vi "ep_Config Info to Task.vi"(6 "trigger timestamp":timestamp, 7 "record info":T1={"station name"="", "recording device name"="", "line frequency [Hz]"=50.0, "timestamp multiplier"=1.0}, 8 "error in (no error)":errorcluster, 9 "status channel info":T10[](array[typedef]), 10 "analog channel info":T11[](array[typedef]), 11 "task in":T2={"file refnums"=[], "Data Object"=refnum, "config info"={"station_name"="", "rec_dev_id"="", "rev_year"=1999.0, "TT"=0, "##A"=0, "##D"=0, "analog channel info"=[], "status channel info"=[], "lf"=-inf, "nrates"=65535, "samp info"=[], "initial timestamp"=timestamp(0 s since 1904-01-01), "trigger timestamp"=timestamp(0 s since 1904-01-01), "ft"=enum."Binary", "timemult"=1.0}, "public inf content"={"Source"="", "Record Type"=enum."Fault", "Phase ID"="", "Event Description"="", "Device ID"="", "Distance of Fault"=-1.0, "Distance Unit"=enum."Miles", "Max_Current"=inf, "Min_Current"=-inf, "Max_Voltage"=inf, "Min_Voltage"=-inf, "EventNoteCount"=0, "Event Information"=[]}, "private inf content"=[], "internal buffers"={"start index"=1, "config to public inf"=enum."disabled", "static config info"="", "static file_des record inf"="", "static file_des channel inf"="", "public inf"="", "private inf"=""}} {"public inf content"."Event Information"."min sample number" max=9999999999; "public inf content"."Event Information"."max sample number" max=9999999999; "config info"."nrates" max=999; "config info"."status channel info"."Dn" min=1 max=999999; "config info"."analog channel info"."An" min=1 max=999999; "config info"."trigger timestamp" format="%<%H:%M:%S%6u\n%d/%m/%Y>T"; "config info"."initial timestamp" format="%<%H:%M:%S%6u\n%d/%m/%Y>T"; "config info"."##D" max=999999; "config info"."##A" max=999999; "config info"."TT" min=1 max=999999; "config info"."rev_year" min=1999.0 max=1999.0}) -> (0 "error out":errorcluster, 3 "task out":T2={"file refnums"=[], "Data Object"=refnum, "config info"={"station_name"="", "rec_dev_id"="", "rev_year"=1999.0, "TT"=0, "##A"=0, "##D"=0, "analog channel info"=[], "status channel info"=[], "lf"=-inf, "nrates"=65535, "samp info"=[], "initial timestamp"=timestamp(0 s since 1904-01-01), "trigger timestamp"=timestamp(0 s since 1904-01-01), "ft"=enum."Binary", "timemult"=1.0}, "public inf content"={"Source"="", "Record Type"=enum."Fault", "Phase ID"="", "Event Description"="", "Device ID"="", "Distance of Fault"=-1.0, "Distance Unit"=enum."Miles", "Max_Current"=inf, "Min_Current"=-inf, "Max_Voltage"=inf, "Min_Voltage"=-inf, "EventNoteCount"=0, "Event Information"=[]}, "private inf content"=[], "internal buffers"={"start index"=1, "config to public inf"=enum."disabled", "static config info"="", "static file_des record inf"="", "static file_des channel inf"="", "public inf"="", "private inf"=""}} {"public inf content"."Event Information"."min sample number" max=9999999999; "public inf content"."Event Information"."max sample number" max=9999999999; "config info"."nrates" max=999; "config info"."status channel info"."Dn" min=1 max=999999; "config info"."analog channel info"."An" min=1 max=999999; "config info"."trigger timestamp" format="%<%H:%M:%S%6u\n%d/%m/%Y>T"; "config info"."initial timestamp" format="%<%H:%M:%S%6u\n%d/%m/%Y>T"; "config info"."##D" max=999999; "config info"."##A" max=999999; "config info"."TT" min=1 max=999999; "config info"."rev_year" min=1999.0 max=1999.0})   [LabVIEW 2011, in "NI_EP_COMTRADE.lvlib"]
uses:
  <vilib>/addons/Electrical Power/File IO/NI_EP_COMTRADE.lvlib
  <vilib>/addons/Electrical Power/File IO/COMTRADE/typedefs/ep_Analog Channel Info (UI).ctl
  <vilib>/addons/Electrical Power/File IO/COMTRADE/typedefs/ep_Status Channel Info (UI).ctl
  <vilib>/addons/Electrical Power/File IO/COMTRADE/typedefs/ep_Task.ctl
  <vilib>/addons/Electrical Power/File IO/COMTRADE/typedefs/ep_Config Info.ctl
  <vilib>/addons/Electrical Power/File IO/COMTRADE/typedefs/ep_Analog Channel Info.ctl
  <vilib>/addons/Electrical Power/File IO/COMTRADE/typedefs/ep_Status Channel Info.ctl
  <vilib>/addons/Electrical Power/File IO/COMTRADE/typedefs/ep_File Format.ctl
  <vilib>/addons/Electrical Power/File IO/COMTRADE/typedefs/ep_Public Inf Content.ctl
  <vilib>/addons/Electrical Power/File IO/COMTRADE/typedefs/ep_Public Event Inf.ctl
  <vilib>/addons/Electrical Power/File IO/COMTRADE/typedefs/ep_Private Inf Content.ctl
  <vilib>/addons/Electrical Power/File IO/COMTRADE/typedefs/ep_System Record Inf.ctl
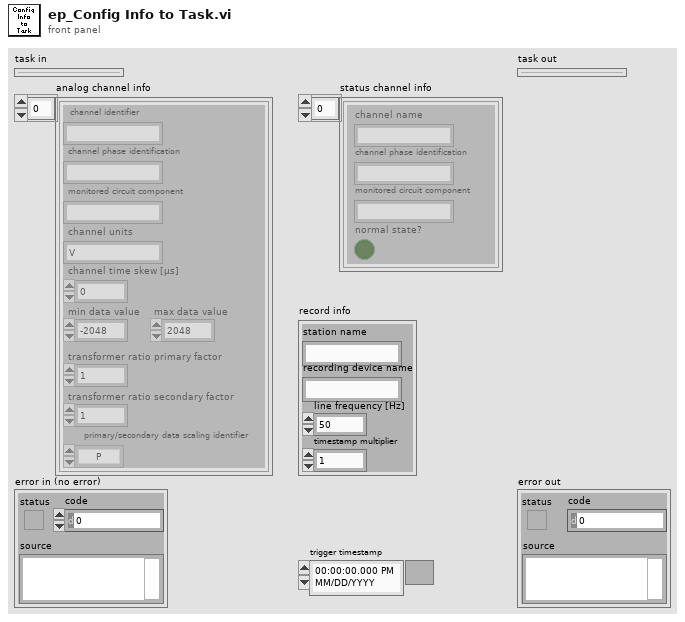
[diagram p1: front panel]
types:
  T1 = typedef "NI_EP_COMTRADE.lvlib/ep_System Record Inf.ctl" = cluster{"station name":string, "recording device name":string, "line frequency [Hz]":sgl, "timestamp multiplier":sgl}
  T2 = typedef "NI_EP_COMTRADE.lvlib/ep_Task.ctl" = cluster{"file refnums":refnum<file>[], "Data Object":refnum<k20>, "config info":T3, "public inf content":T7, "private inf content":T9, "internal buffers":cluster{"start index":u32, "config to public inf":enum16{"disabled", "enabled", "buffered"}, "static config info":string, "static file_des record inf":string, "static file_des channel inf":string, "public inf":string, "private inf":string}}
  T3 = typedef "NI_EP_COMTRADE.lvlib/ep_Config Info.ctl" = cluster{"station_name":string, "rec_dev_id":string, "rev_year":dbl, "TT":u32, "##A":u32, "##D":u32, "analog channel info":T4[], "status channel info":T5[], "lf":sgl, "nrates":u16, "samp info":cluster{"samp":sgl, "endsamp":u32}[], "initial timestamp":timestamp, "trigger timestamp":timestamp, "ft":T6, "timemult":sgl}
  T4 = typedef "NI_EP_COMTRADE.lvlib/ep_Analog Channel Info.ctl" = cluster{"An":u32, "ch_id":string, "ph":string, "ccbm":string, "uu":string, "a":sgl, "b":sgl, "skew":sgl, "min":i32, "max":i32, "primary":sgl, "secondary":sgl, "PS":enum16{"P", "S"}}
  T5 = typedef "NI_EP_COMTRADE.lvlib/ep_Status Channel Info.ctl" = cluster{"Dn":u32, "ch_id":string, "ph":string, "ccbm":string, "Y":bool}
  T6 = typedef "NI_EP_COMTRADE.lvlib/ep_File Format.ctl" = enum16{"ASCII", "Binary"}
  T7 = typedef "NI_EP_COMTRADE.lvlib/ep_Public Inf Content.ctl" = cluster{"Source":string, "Record Type":enum16{"Fault", "Unknown", "Misoperation", "Close", "Trip", "Reclose", "Power swing", "Simulation"}, "Phase ID":string, "Event Description":string, "Device ID":string, "Distance of Fault":dbl, "Distance Unit":enum16{"Miles", "Kilometers", "Percent of line", "Percent of setting", "Ohms"}, "Max_Current":dbl, "Min_Current":dbl, "Max_Voltage":dbl, "Min_Voltage":dbl, "EventNoteCount":u32, "Event Information":T8[]}
  T8 = typedef "NI_EP_COMTRADE.lvlib/ep_Public Event Inf.ctl" = cluster{"channel number":u32, "max value":dbl, "min value":dbl, "max sample number":u64, "min sample number":u64, "max sample text":string[], "min sample text":string[]}
  T9 = typedef "NI_EP_COMTRADE.lvlib/ep_Private Inf Content.ctl" = cluster{"Section Header":string, "Entry Names":string[], "Entry Values":string[]}[]
  T10 = typedef "NI_EP_COMTRADE.lvlib/ep_Status Channel Info (UI).ctl" = cluster{"channel name":string, "channel phase identification":string, "monitored circuit component":string, "normal state?":bool}
  T11 = typedef "NI_EP_COMTRADE.lvlib/ep_Analog Channel Info (UI).ctl" = cluster{"channel identifier":string, "channel phase identification":string, "monitored circuit component":string, "channel units":string, "channel time skew [µs]":sgl, "min data value":sgl, "max data value":sgl, "transformer ratio primary factor":sgl, "transformer ratio secondary factor":sgl, "primary/secondary data scaling identifier":enum16{"P", "S"}}
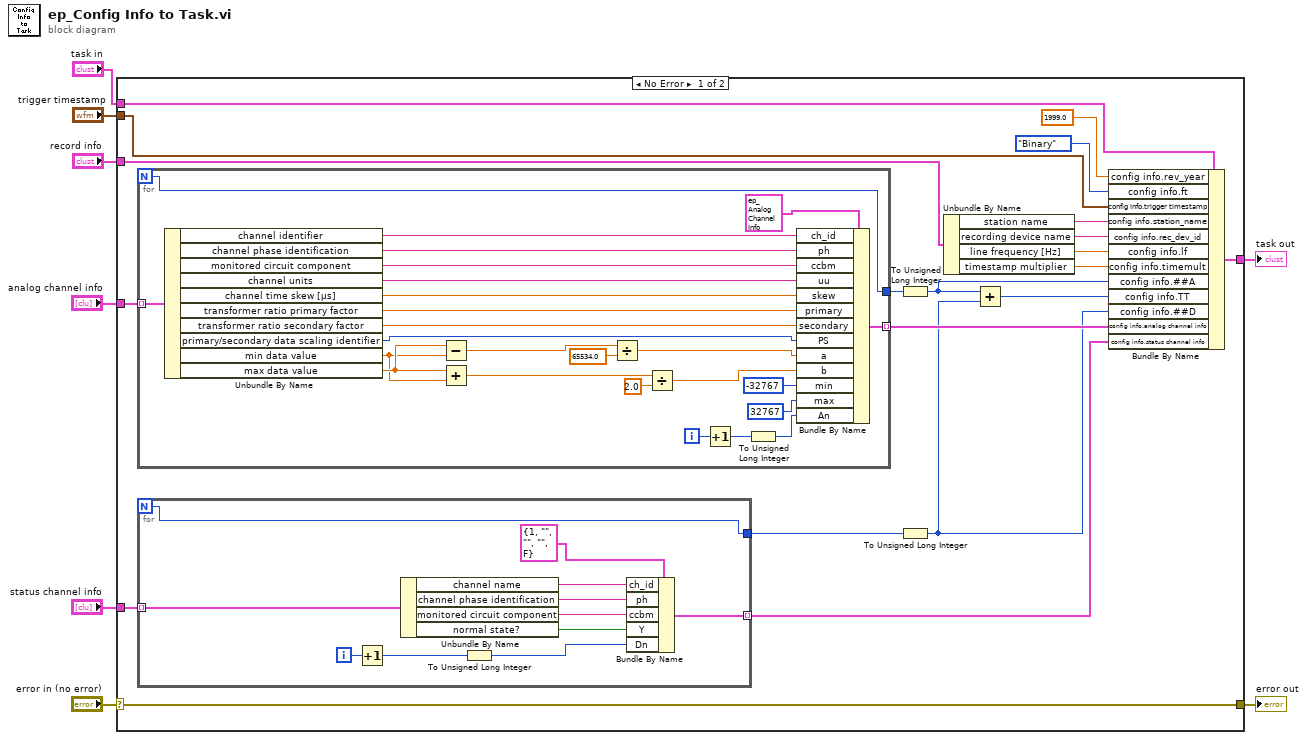
[diagram p0: block diagram]
diagram:
  n1 = case shown="No Error" "error in (no error)" {
    selector: "error in (no error)" -> [w28 w66]
    tunnel: [w28 w66] -> w7
    tunnel: "record info" -> [w26 _]
    tunnel: "analog channel info" -> [w20 _]
    tunnel: "status channel info" -> [w23 _]
    tunnel: [w27 w65] -> w4
    tunnel: "trigger timestamp" -> [w18 _]
    tunnel: "task in" -> [w17 w65]
    frame No Error {
      n2 = for {
        N -> [w53]
        tunnel: w20 -> [w52] mode=indexing
        tunnel: [w53] -> w15
        tunnel: [w39] -> w19 mode=indexing
        i -> [w40]
        n3 = Unbundle By Name(w52) -> ("channel identifier"=w51:string, "channel phase identification"=w50:string, "monitored circuit component"=w49:string, "channel units"=w48:string, "channel time skew [µs]"=w33:sgl, "transformer ratio primary factor"=w32:sgl, "transformer ratio secondary factor"=w31:sgl, "primary/secondary data scaling identifier"=w47:enum16{"P", "S"}, "min data value"=w43:sgl, "max data value"=w44:sgl)
        n4 = Subtract(x=w44, y=w43) -> (x-y=w46:sgl)
        n5 = Add(x=w44, y=w43) -> (x+y=w42:sgl)
        n6 = Divide(x=w46, y=sgl 65534.0) -> (x/y=w30:sgl)
        n7 = Divide(x=w42, y=sgl 2.0) -> (x/y=w29:sgl)
        n8 = Increment(x=w40) -> (x+1=w36:i32)
        n9 = To Unsigned Long Integer(number=w36) -> (unsigned 32bit integer=w35:u32)
        n10 = Bundle By Name(cluster=T4 {"An"=1, "ch_id"="", "ph"="", "ccbm"="", "uu"="V", "a"=0.0, "b"=0.0, "skew"=0.0, "min"=-32767, "max"=32767, "primary"=1.0, "secondary"=1.0, "PS"=enum."P"} ("element"), "ch_id"=w51, "ph"=w50, "ccbm"=w49, "uu"=w48, "skew"=w33, "primary"=w32, "secondary"=w31, "PS"=w47, "a"=w30, "b"=w29, "min"=-32767, "max"=32767, "An"=w35) -> (w39:T4)
      }
      n11 = for {
        N -> [w58]
        tunnel: w23 -> [w64] mode=indexing
        tunnel: [w59] -> w22 mode=indexing
        tunnel: [w58] -> w16
        i -> [w57]
        n12 = Increment(x=w57) -> (x+1=w56:i32)
        n13 = Unbundle By Name(w64) -> ("channel name"=w63:string, "channel phase identification"=w62:string, "monitored circuit component"=w61:string, "normal state?"=w60:bool)
        n14 = To Unsigned Long Integer(number=w56) -> (unsigned 32bit integer=w55:u32)
        n15 = Bundle By Name(cluster=T5 {"Dn"=1, "ch_id"="", "ph"="", "ccbm"="", "Y"=FALSE} ("element"), "ch_id"=w63, "ph"=w62, "ccbm"=w61, "Y"=w60, "Dn"=w55) -> (w59:T5)
      }
      n16 = To Unsigned Long Integer(number=w15) -> (unsigned 32bit integer=w14:u32)
      n17 = To Unsigned Long Integer(number=w16) -> (unsigned 32bit integer=w13:u32)
      n18 = Unbundle By Name(w26) -> ("station name"=w25:string, "recording device name"=w24:string, "line frequency [Hz]"=w12:sgl, "timestamp multiplier"=w11:sgl)
      n19 = Add(x=w14, y=w13) -> (x+y=w21:u32)
      n20 = Bundle By Name(cluster=w17, "config info.rev_year"=1999.0, "config info.ft"=ep_File_Format."Binary", "config info.trigger timestamp"=w18, "config info.station_name"=w25, "config info.rec_dev_id"=w24, "config info.lf"=w12, "config info.timemult"=w11, "config info.##A"=w14, "config info.TT"=w21, "config info.##D"=w13, "config info.analog channel info"=w19, "config info.status channel info"=w22) -> (w27:T2)
    }
    frame Error {
    }
  }
  "error out" <- w7
  "task out" <- w4
